vi "_RUN_HVAC_PROJECT.vi"() -> ()   [LabVIEW 2011]
panel:
  in  "Tab Control":T1(tab)
  in  "Stop":bool
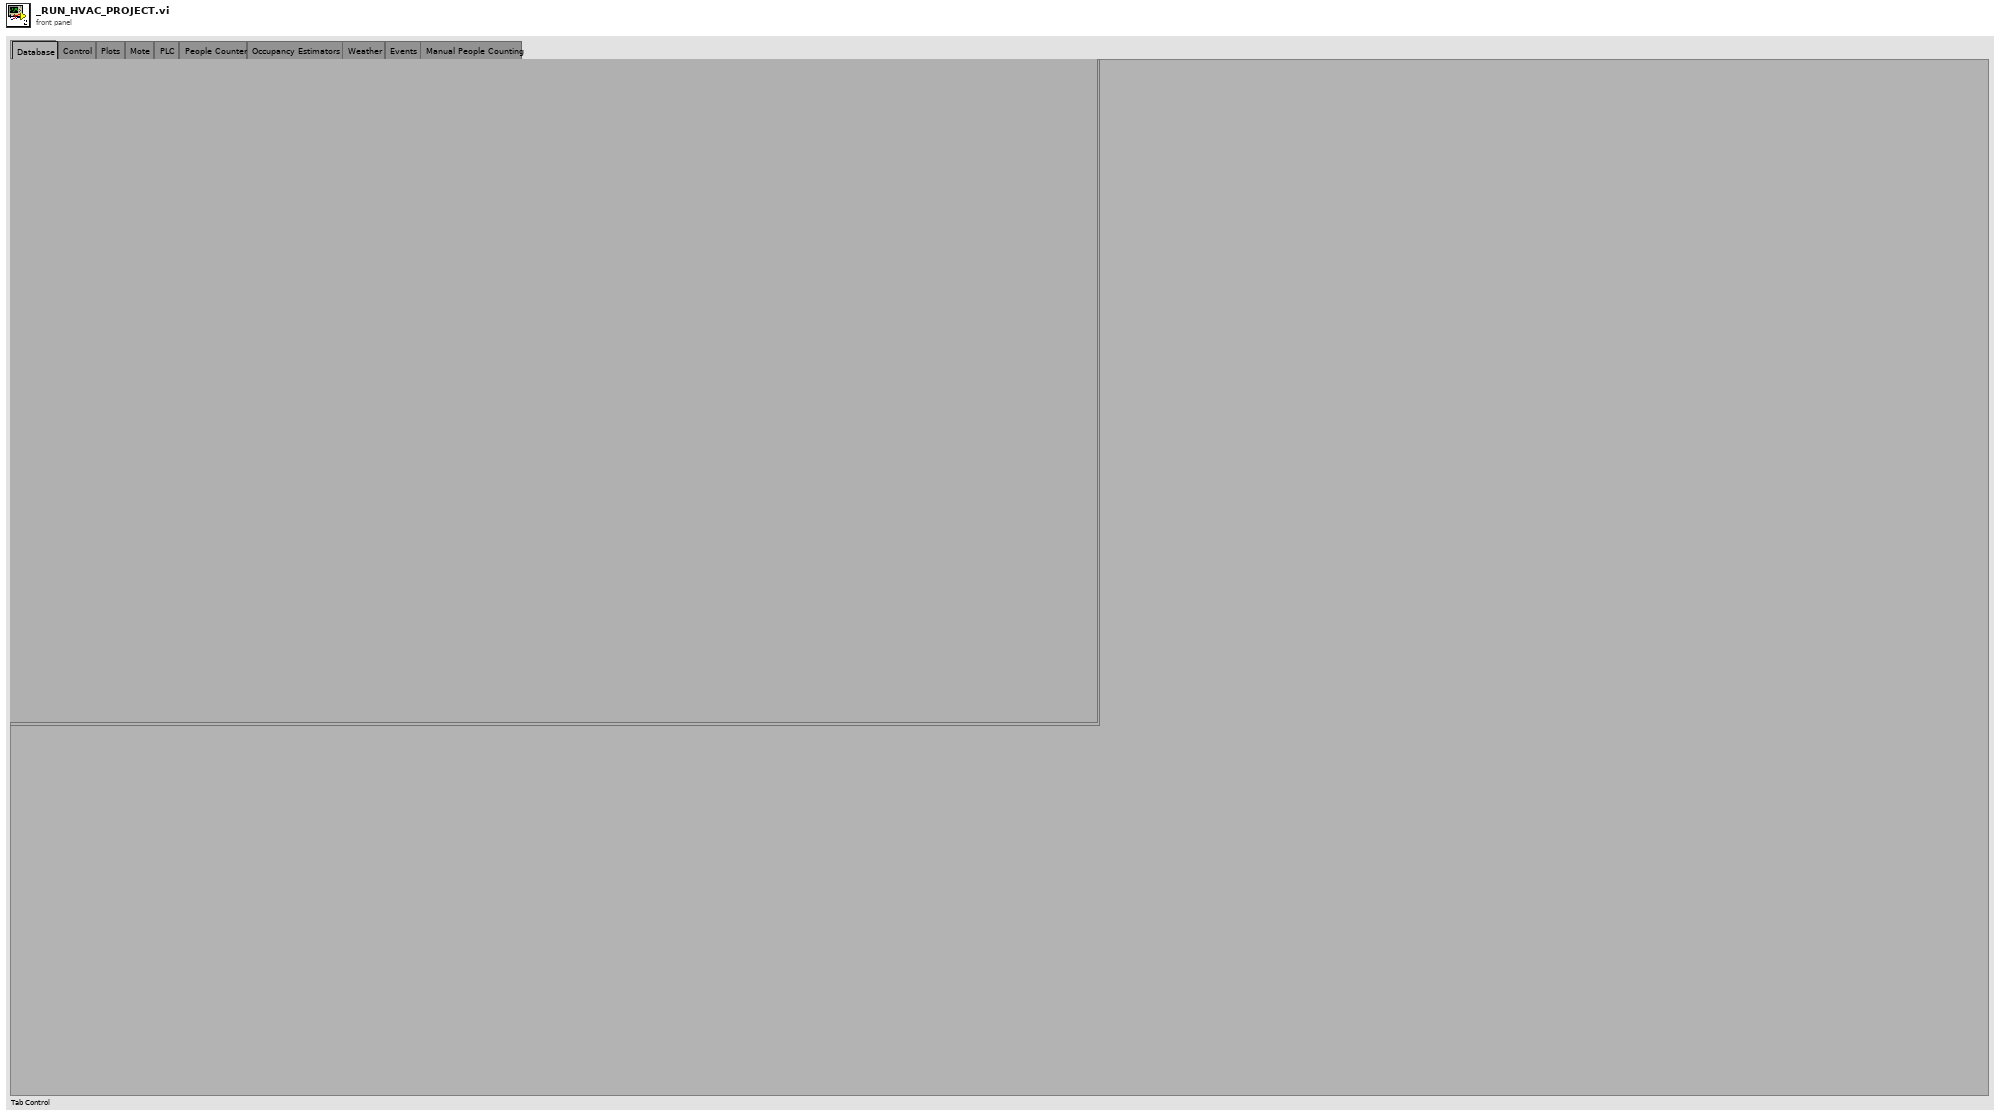
[diagram p1: front panel]
types:
  T1 = enum32{"Database", "Control", "Plots", "Mote", "PLC", "People Counter", "Occupancy Estimators", "Weather", "Events", "Manual People Counting"}
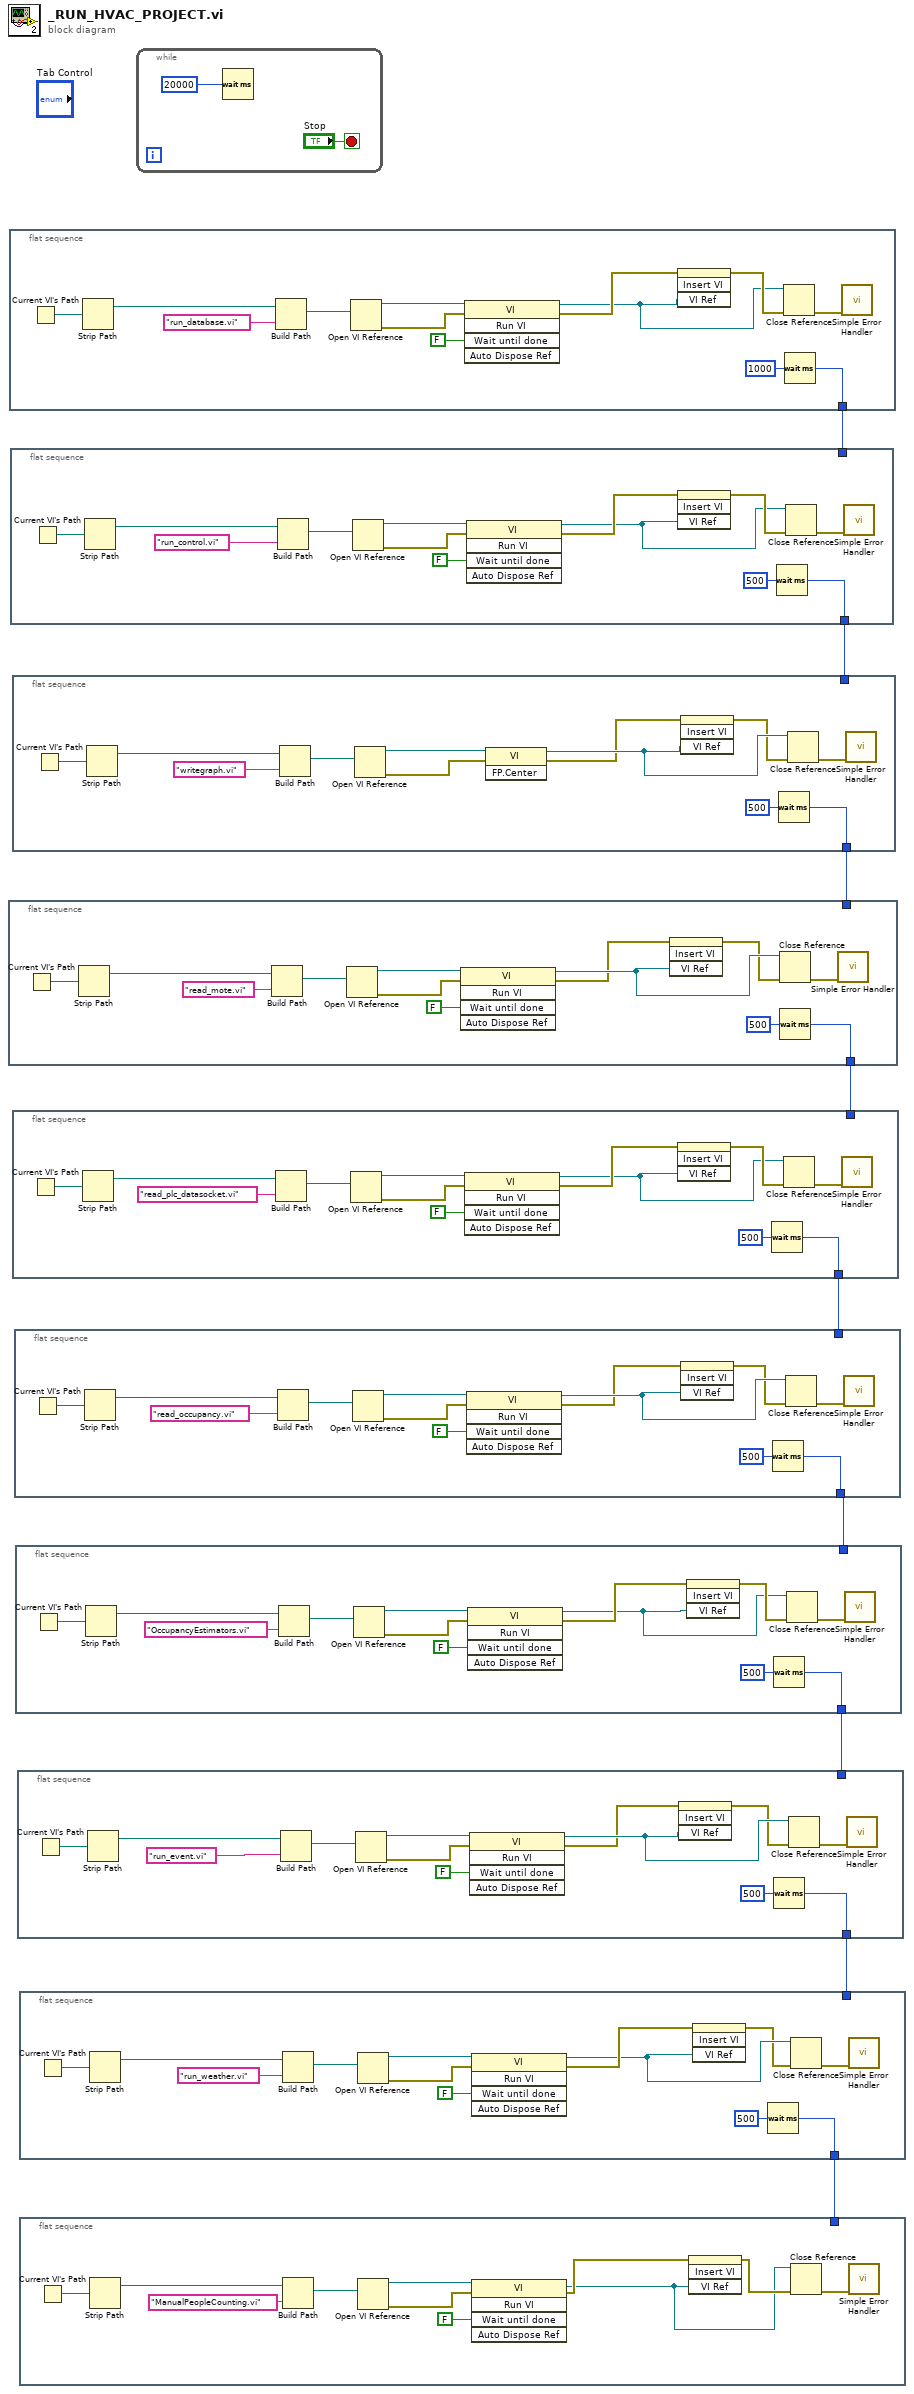
[diagram p0: block diagram]
diagram:
  n1 = flat-sequence {
    tunnel: [w10] -> w8
    tunnel: w4 -> [_]
    frame #0 {
      n2 = Current VI's Path() -> (path=w19:path)
      n3 = Strip Path(path=w19) -> (stripped path=w17:path)  [unwired: 1 out]
      n4 = Build Path(base path=w17, name or relative path="read_mote.vi") -> (appended path=w18:path)
      n5 = Open VI Reference(vi path=w18) -> (vi reference=w22:refnum<vi>, error out=w21:errorcluster)  [unwired: 5 in]
      n6 = invoke class="VI" method="Run VI"(reference=w22, error in=w21, "Wait until done"=FALSE) -> (reference out=w14:refnum<vi>, error out=w13:errorcluster)  [unwired: 2 in, 3 out]
      n7 = invoke class="SubPanel" method="Insert VI"(error in=w13, "VI Ref"=w14) -> (error out=w12:errorcluster)  [unwired: 2 in, 3 out]
      n8 = Close Reference(reference=w14, error in (no error)=w12) -> (error out=w16:errorcluster)
      n9 = Wait (ms)(milliseconds to wait=u32 500) -> (millisecond timer value=w10:u32)
      n10 = call <vilib>:"Simple Error Handler.vi"("error in (no error)"=w16) -> ()  [unwired: 4 in, 5 out]
    }
  }
  n11 = flat-sequence {
    tunnel: [w23] -> w9
    frame #0 {
      n12 = Current VI's Path() -> (path=w32:path)
      n13 = Strip Path(path=w32) -> (stripped path=w30:path)  [unwired: 1 out]
      n14 = Build Path(base path=w30, name or relative path="run_database.vi") -> (appended path=w31:path)
      n15 = Open VI Reference(vi path=w31) -> (vi reference=w35:refnum<vi>, error out=w34:errorcluster)  [unwired: 5 in]
      n16 = invoke class="VI" method="Run VI"(reference=w35, error in=w34, "Wait until done"=FALSE) -> (reference out=w25:refnum<vi>, error out=w26:errorcluster)  [unwired: 2 in, 3 out]
      n17 = invoke class="SubPanel" method="Insert VI"(error in=w26, "VI Ref"=w25) -> (error out=w27:errorcluster)  [unwired: 2 in, 3 out]
      n18 = Close Reference(reference=w25, error in (no error)=w27) -> (error out=w29:errorcluster)
      n19 = Wait (ms)(milliseconds to wait=u32 1000) -> (millisecond timer value=w23:u32)
      n20 = call <vilib>:"Simple Error Handler.vi"("error in (no error)"=w29) -> ()  [unwired: 4 in, 5 out]
    }
  }
  n21 = flat-sequence {
    tunnel: w9 -> [_]
    tunnel: [w36] -> w5
    frame #0 {
      n22 = Current VI's Path() -> (path=w44:path)
      n23 = Strip Path(path=w44) -> (stripped path=w46:path)  [unwired: 1 out]
      n24 = Build Path(base path=w46, name or relative path="run_control.vi") -> (appended path=w45:path)
      n25 = Open VI Reference(vi path=w45) -> (vi reference=w41:refnum<vi>, error out=w42:errorcluster)  [unwired: 5 in]
      n26 = invoke class="VI" method="Run VI"(reference=w41, error in=w42, "Wait until done"=FALSE) -> (reference out=w38:refnum<vi>, error out=w39:errorcluster)  [unwired: 2 in, 3 out]
      n27 = invoke class="SubPanel" method="Insert VI"(error in=w39, "VI Ref"=w38) -> (error out=w40:errorcluster)  [unwired: 2 in, 3 out]
      n28 = Wait (ms)(milliseconds to wait=u32 500) -> (millisecond timer value=w36:u32)
      n29 = Close Reference(reference=w38, error in (no error)=w40) -> (error out=w47:errorcluster)
      n30 = call <vilib>:"Simple Error Handler.vi"("error in (no error)"=w47) -> ()  [unwired: 4 in, 5 out]
    }
  }
  n31 = flat-sequence {
    tunnel: [w52] -> w4
    tunnel: w5 -> [_]
    frame #0 {
      n32 = Current VI's Path() -> (path=w56:path)
      n33 = Strip Path(path=w56) -> (stripped path=w58:path)  [unwired: 1 out]
      n34 = Build Path(base path=w58, name or relative path="writegraph.vi") -> (appended path=w57:path)
      n35 = Open VI Reference(vi path=w57) -> (vi reference=w54:refnum<vi>, error out=w55:errorcluster)  [unwired: 5 in]
      n36 = invoke class="VI" method="FP.Center"(reference=w54, error in=w55) -> (reference out=w51:refnum<vi>, error out=w50:errorcluster)  [unwired: 1 in, 1 out]
      n37 = invoke class="SubPanel" method="Insert VI"(error in=w50, "VI Ref"=w51) -> (error out=w49:errorcluster)  [unwired: 2 in, 3 out]
      n38 = Wait (ms)(milliseconds to wait=u32 500) -> (millisecond timer value=w52:u32)
      n39 = Close Reference(reference=w51, error in (no error)=w49) -> (error out=w59:errorcluster)
      n40 = call <vilib>:"Simple Error Handler.vi"("error in (no error)"=w59) -> ()  [unwired: 4 in, 5 out]
    }
  }
  n41 = flat-sequence {
    tunnel: w8 -> [_]
    tunnel: [w61] -> w7
    frame #0 {
      n42 = Current VI's Path() -> (path=w69:path)
      n43 = Strip Path(path=w69) -> (stripped path=w71:path)  [unwired: 1 out]
      n44 = Build Path(base path=w71, name or relative path="read_plc_datasocket.vi") -> (appended path=w70:path)
      n45 = Open VI Reference(vi path=w70) -> (vi reference=w66:refnum<vi>, error out=w67:errorcluster)  [unwired: 5 in]
      n46 = invoke class="VI" method="Run VI"(reference=w66, error in=w67, "Wait until done"=FALSE) -> (reference out=w63:refnum<vi>, error out=w64:errorcluster)  [unwired: 2 in, 3 out]
      n47 = invoke class="SubPanel" method="Insert VI"(error in=w64, "VI Ref"=w63) -> (error out=w65:errorcluster)  [unwired: 2 in, 3 out]
      n48 = Wait (ms)(milliseconds to wait=u32 500) -> (millisecond timer value=w61:u32)
      n49 = Close Reference(reference=w63, error in (no error)=w65) -> (error out=w72:errorcluster)
      n50 = call <vilib>:"Simple Error Handler.vi"("error in (no error)"=w72) -> ()  [unwired: 4 in, 5 out]
    }
  }
  n51 = flat-sequence {
    tunnel: w7 -> [_]
    tunnel: [w74] -> w2
    frame #0 {
      n52 = Current VI's Path() -> (path=w82:path)
      n53 = Strip Path(path=w82) -> (stripped path=w84:path)  [unwired: 1 out]
      n54 = Build Path(base path=w84, name or relative path="read_occupancy.vi") -> (appended path=w83:path)
      n55 = Open VI Reference(vi path=w83) -> (vi reference=w79:refnum<vi>, error out=w80:errorcluster)  [unwired: 5 in]
      n56 = invoke class="VI" method="Run VI"(reference=w79, error in=w80, "Wait until done"=FALSE) -> (reference out=w78:refnum<vi>, error out=w77:errorcluster)  [unwired: 2 in, 3 out]
      n57 = invoke class="SubPanel" method="Insert VI"(error in=w77, "VI Ref"=w78) -> (error out=w76:errorcluster)  [unwired: 2 in, 3 out]
      n58 = Wait (ms)(milliseconds to wait=u32 500) -> (millisecond timer value=w74:u32)
      n59 = Close Reference(reference=w78, error in (no error)=w76) -> (error out=w85:errorcluster)
      n60 = call <vilib>:"Simple Error Handler.vi"("error in (no error)"=w85) -> ()  [unwired: 4 in, 5 out]
    }
  }
  n61 = flat-sequence {
    tunnel: [w91] -> w1
    tunnel: [w87] -> _
    tunnel: w2 -> [w87]
    frame #0 {
      n62 = Current VI's Path() -> (path=w96:path)
      n63 = Strip Path(path=w96) -> (stripped path=w98:path)  [unwired: 1 out]
      n64 = Build Path(base path=w98, name or relative path="OccupancyEstimators.vi") -> (appended path=w97:path)
      n65 = Open VI Reference(vi path=w97) -> (vi reference=w93:refnum<vi>, error out=w94:errorcluster)  [unwired: 5 in]
      n66 = invoke class="VI" method="Run VI"(reference=w93, error in=w94, "Wait until done"=FALSE) -> (reference out=w88:refnum<vi>, error out=w89:errorcluster)  [unwired: 2 in, 3 out]
      n67 = invoke class="SubPanel" method="Insert VI"(error in=w89, "VI Ref"=w88) -> (error out=w90:errorcluster)  [unwired: 2 in, 3 out]
      n68 = Wait (ms)(milliseconds to wait=u32 500) -> (millisecond timer value=w91:u32)
      n69 = Close Reference(reference=w88, error in (no error)=w90) -> (error out=w99:errorcluster)
      n70 = call <vilib>:"Simple Error Handler.vi"("error in (no error)"=w99) -> ()  [unwired: 4 in, 5 out]
    }
  }
  n71 = flat-sequence {
    tunnel: [w101] -> w6
    tunnel: w1 -> [_]
    frame #0 {
      n72 = Current VI's Path() -> (path=w109:path)
      n73 = Strip Path(path=w109) -> (stripped path=w111:path)  [unwired: 1 out]
      n74 = Build Path(base path=w111, name or relative path="run_event.vi") -> (appended path=w110:path)
      n75 = Open VI Reference(vi path=w110) -> (vi reference=w106:refnum<vi>, error out=w107:errorcluster)  [unwired: 5 in]
      n76 = invoke class="VI" method="Run VI"(reference=w106, error in=w107, "Wait until done"=FALSE) -> (reference out=w105:refnum<vi>, error out=w104:errorcluster)  [unwired: 2 in, 3 out]
      n77 = invoke class="SubPanel" method="Insert VI"(error in=w104, "VI Ref"=w105) -> (error out=w103:errorcluster)  [unwired: 2 in, 3 out]
      n78 = Wait (ms)(milliseconds to wait=u32 500) -> (millisecond timer value=w101:u32)
      n79 = Close Reference(reference=w105, error in (no error)=w103) -> (error out=w112:errorcluster)
      n80 = call <vilib>:"Simple Error Handler.vi"("error in (no error)"=w112) -> ()  [unwired: 4 in, 5 out]
    }
  }
  n81 = flat-sequence {
    tunnel: w6 -> [_]
    tunnel: [w114] -> w3
    frame #0 {
      n82 = Current VI's Path() -> (path=w122:path)
      n83 = Strip Path(path=w122) -> (stripped path=w124:path)  [unwired: 1 out]
      n84 = Build Path(base path=w124, name or relative path="run_weather.vi") -> (appended path=w123:path)
      n85 = Open VI Reference(vi path=w123) -> (vi reference=w119:refnum<vi>, error out=w120:errorcluster)  [unwired: 5 in]
      n86 = invoke class="VI" method="Run VI"(reference=w119, error in=w120, "Wait until done"=FALSE) -> (reference out=w117:refnum<vi>, error out=w118:errorcluster)  [unwired: 2 in, 3 out]
      n87 = invoke class="SubPanel" method="Insert VI"(error in=w118, "VI Ref"=w117) -> (error out=w116:errorcluster)  [unwired: 2 in, 3 out]
      n88 = Wait (ms)(milliseconds to wait=u32 500) -> (millisecond timer value=w114:u32)
      n89 = Close Reference(reference=w117, error in (no error)=w116) -> (error out=w125:errorcluster)
      n90 = call <vilib>:"Simple Error Handler.vi"("error in (no error)"=w125) -> ()  [unwired: 4 in, 5 out]
    }
  }
  n91 = flat-sequence {
    tunnel: w3 -> [_]
    frame #0 {
      n92 = Current VI's Path() -> (path=w133:path)
      n93 = Strip Path(path=w133) -> (stripped path=w135:path)  [unwired: 1 out]
      n94 = Build Path(base path=w135, name or relative path="ManualPeopleCounting.vi") -> (appended path=w134:path)
      n95 = Open VI Reference(vi path=w134) -> (vi reference=w130:refnum<vi>, error out=w131:errorcluster)  [unwired: 5 in]
      n96 = invoke class="VI" method="Run VI"(reference=w130, error in=w131, "Wait until done"=FALSE) -> (reference out=w127:refnum<vi>, error out=w129:errorcluster)  [unwired: 2 in, 3 out]
      n97 = invoke class="SubPanel" method="Insert VI"(error in=w129, "VI Ref"=w127) -> (error out=w128:errorcluster)  [unwired: 2 in, 3 out]
      n98 = Close Reference(reference=w127, error in (no error)=w128) -> (error out=w136:errorcluster)
      n99 = call <vilib>:"Simple Error Handler.vi"("error in (no error)"=w136) -> ()  [unwired: 4 in, 5 out]
    }
  }
  n100 = while {
    stop <- "Stop" stop-if-true
    n101 = Wait (ms)(milliseconds to wait=u32 20000) -> ()  [unwired: 1 out]
  }
